vi "Tosca-Masker Thread.vi"(7 "IPC":T1, 11 "Tosca":refnum<class "Parameters.lvclass">) -> (0 "error out":errorcluster)   [LabVIEW 2020]
uses:
  IPC VIs/Tosca-IPC.ctl
  Classes/Parameters/Parameters.lvclass
  Digital Input VIs/Tosca-DI Queue Data.ctl
  Digital Input VIs/Tosca-Input Event.ctl
  Digital Input VIs/Tosca-Input Criterion.ctl
  epl-vi-lib/Utility VIs/Type Defs/Logic State.ctl
  Typedefs/Tosca-Accumulator.ctl
  Typedefs/Tosca-State AODO.ctl
  Typedefs/Tosca-AO Runtime.ctl
  Typedefs/Tosca-DO Runtime.ctl
  epl-vi-lib/Signal Synthesis VIs/4th Generation/Classes/SignalManager/SignalManager.lvclass
  Typedefs/Tosca-Synapse Start Data.ctl
  IPC VIs/Tosca-Message.ctl
  IPC VIs/Tosca-Message Action.ctl
  Typedefs/Tosca-Thread Type.ctl
  Imaging VIs/Tosca-2P-Notifier Data.ctl
  Typedefs/Tosca-MATLAB Queue Data.ctl
  Visual Stim VIs/Tosca-Grating.ctl
  Visual Stim VIs/Tosca-Grating Type.ctl
  Typedefs/Tosca-File IO Notification.ctl
  Classes/Parameters/Parameters.lvclass/Parameters.ctl
  epl-vi-lib/Signal Synthesis VIs/4th Generation/Classes/Channel/Channel.lvclass/Channel.ctl
  epl-vi-lib/Signal Synthesis VIs/4th Generation/Classes/Level/Level.lvclass/Level.ctl
  05e3e8bd-c3cb-450d-bf27-de7c8e806e93.vi
  9dbdce7e-9137-4943-9ff0-cc94a39cad21.vi
  epl-vi-lib/Signal Synthesis VIs/4th Generation/Classes/Channel/Write Level Value.vi
  <vilib>/DAQmx/write.llb/DAQmx Write (Analog 1D DBL 1Chan NSamp).vi
  epl-vi-lib/Signal Synthesis VIs/4th Generation/Classes/Channel/Read Destination.vi
  Classes/Parameters/Read Use masker.vi
  Classes/Parameters/Read Masker.vi
  Classes/Parameters/Read DAQ.vi
  epl-vi-lib/Signal Synthesis VIs/4th Generation/Classes/Level/Write Level.vi
  epl-vi-lib/Utility VIs/Controls/Utilities-Wait.vi/89bc9713-8f2c-40bd-a11f-1c800a437687.vi
  Tosca-Globals.vi
  <vilib>/Utility/config.llb/Open Config Data.vi
  <vilib>/Utility/config.llb/Get Key Names.vi
  <vilib>/Utility/config.llb/Read Key.vi
  <vilib>/Utility/config.llb/Read Key (String).vi
  epl-vi-lib/Utility VIs/Array Manipulation VIs/String Array to Comma Separated String.vi
  <vilib>/Utility/error.llb/Error Cluster From Error Code.vi
  <vilib>/Utility/config.llb/Close Config Data.vi
  <vilib>/DAQmx/miscellaneous.llb/DAQmx Fill In Error Info.vi
  <vilib>/Utility/High Resolution Polling Wait.vi
  epl-vi-lib/Signal Synthesis VIs/4th Generation/Classes/Channel/Channel.lvclass
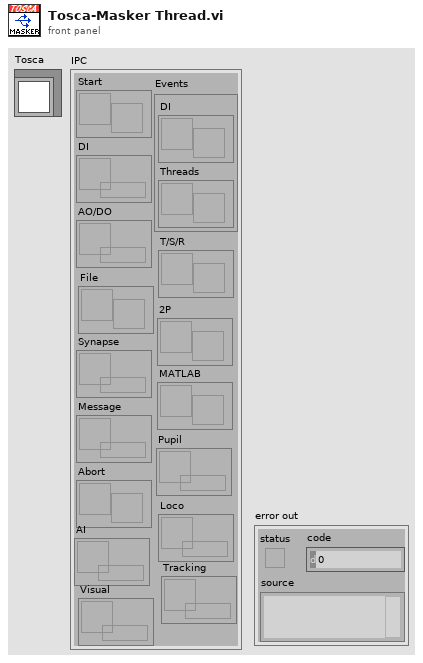
[diagram p1: front panel]
types:
  T1 = typedef "Tosca-IPC.ctl" = cluster{"Start":refnum<notifier>, "DI":refnum<queue>, "AO/DO":refnum<queue>, "Synapse":refnum<queue>, "Message":refnum<queue>, "Abort":refnum<notifier>, "Events":cluster{"DI":refnum<user-event>, "Threads ":refnum<user-event>}, "T/S/R":refnum<notifier>, "2P":refnum<notifier>, "MATLAB":refnum<notifier>, "Pupil":refnum<queue>, "Loco":refnum<queue>, "AI":refnum<queue>, "Tracking":refnum<queue>, "Visual":refnum<queue>, "File":refnum<notifier>}
  T2 = typedef "Parameters.lvclass/DAQ.ctl" = cluster{"AO Fs (Hz)":dbl, "DO Fs (Hz)":dbl, "Poll Rate (Hz)":dbl, "Baseline (s)":dbl}
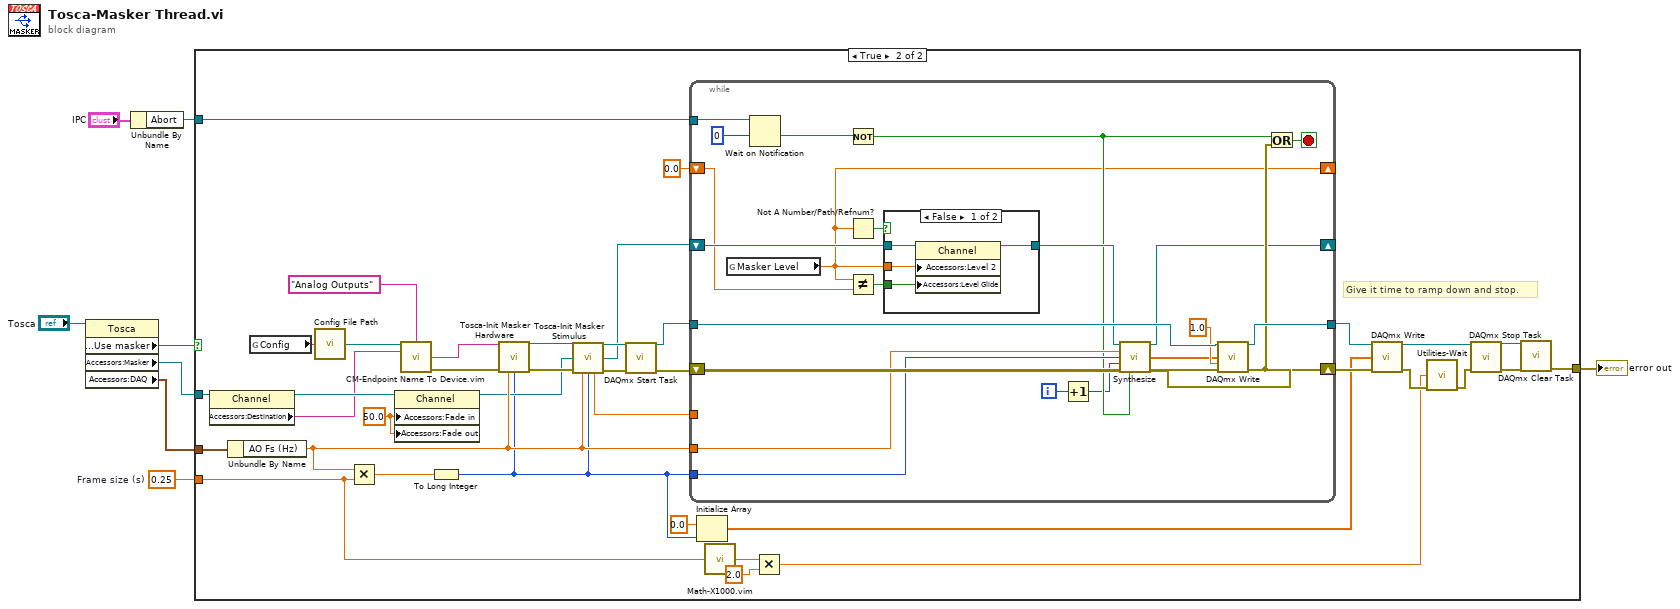
[diagram p0: block diagram]
diagram:
  w8 = 0.25  # Frame size (s)
  n1 = property class="Tosca"(reference="Tosca") -> ("Accessors:Use masker"=w3:bool, "Accessors:Masker"=w2:refnum<class "Channel.lvclass">, "Accessors:DAQ"=w1:T2)  [unwired: 1 in, 2 out]
  n2 = Unbundle By Name("IPC") -> ("Abort"=w5:refnum<notifier>)
  n3 = case shown="True" w3 {
    tunnel: w8 -> [_ w12]
    tunnel: [_ w37] -> w7
    tunnel: w5 -> [_ w35]
    tunnel: w2 -> [_ w33]
    tunnel: w1 -> [_ w32]
    frame False {
    }
    frame True {
      w27 = 50.0 ("Fade in")
      # "Give it time to ramp down and stop."
      n4 = property class="Channel"(reference=w33) -> (reference out=w30:refnum<class "Channel.lvclass">, "Accessors:Destination"=w24:string)  [unwired: 1 in, 1 out]
      n5 = Unbundle By Name(w32) -> ("AO Fs (Hz)"=w31:dbl)
      n6 = global read "Tosca-Globals.vi" "Config"() -> (w34:string)
      n7 = call "Config File Path.vi"("AppName"=w34) -> ("Default config file name"=w26:path)
      n8 = Multiply(x=w31, y=w12) -> (x*y=w46:dbl)
      n9 = property class="Channel"(reference=w30, "Accessors:Fade in"=w27, "Accessors:Fade out"=w27) -> (reference out=w28:refnum<class "Channel.lvclass">)  [unwired: 1 in, 1 out]
      n10 = call "CM-Endpoint Name To Device.vim"("Path"=w26, "IO Type"="Analog Outputs", "Names in"=w24) -> ("Devices"=w23:string, "error out"=w25:errorcluster)  [unwired: 9 in, 2 out]
      n11 = To Long Integer(number=w46) -> (32bit integer=w17:i32)
      n12 = call "Tosca-Init Masker Hardware.vi"("Channel"=w23, "error in (no error)"=w25, "Sampling rate (Hz)"=w31, "Npts"=w17) -> ("task out"=w44:refnum<k21>, "error out"=w45:errorcluster)  [unwired: 10 in]
      n13 = call "Tosca-Init Masker Stimulus.vi"("task in"=w44, "Channel"=w28, "error in (no error)"=w45, "Sampling rate (Hz)"=w31, "Npts"=w17) -> ("task out"=w36:refnum<k21>, "Channel out"=w29:refnum<class "Channel.lvclass">, "Ramp (ms)"=w38:dbl, "error out"=w39:errorcluster)  [unwired: 7 in]
      n14 = call <vilib>:"DAQmx Start Task.vi"("task/channels in"=w36, "error in"=w39) -> ("task out"=w40:refnum<k21>, "error out"=w41:errorcluster)  [unwired: 12 in]
      n15 = while {
        tunnel: w40 -> [w65]
        tunnel: [w67] -> w19
        shift-right: [w59] -> _
        shift-left: w29 -> [w68]
        tunnel: w31 -> [w55]
        tunnel: w17 -> [w56]
        tunnel: w38 -> [_]
        tunnel: w35 -> [w60]
        shift-right: [w62] -> w20
        shift-left: w41 -> [w69]
        shift-right: [w49] -> _
        shift-left: 0.0 ("Masker Level") -> [w50]
        i -> [w51]
        stop <- w66 stop-if-true
        n16 = global read "Tosca-Globals.vi" "Masker Level"() -> (w49:dbl)
        n17 = Wait on Notification(notifier=w60, timeout in ms (-1)=0) -> (timed out?=w53:bool)  [unwired: 2 in, 3 out]
        n18 = Not(x=w53) -> (.not. x?=w52:bool)
        n19 = Not A Number/Path/Refnum?(number/path/refnum=w49) -> (NaN/Path/Refnum?=w61:bool)
        n20 = Not Equal?(x=w49, y=w50) -> (x != y?=w48:bool)
        n21 = case shown="False" w61 {
          tunnel: w68 -> [w73 w74]
          tunnel: [w72 w74] -> w58
          tunnel: w49 -> [w71 _]
          tunnel: w48 -> [w70 _]
          frame False {
            n22 = property class="Channel"(reference=w73, "Accessors:Level 2"=w71, "Accessors:Level Glide"=w70) -> (reference out=w72:refnum<class "Channel.lvclass">)  [unwired: 1 in, 1 out]
          }
          frame True {
          }
        }
        n23 = Increment(x=w51) -> (x+1=w47:i32)
        n24 = call "Synthesize.vi"("Channel in"=w58, "Fs (Hz)"=w55, "Npts"=w56, "Repetition"=w47, "error in (no error)"=w69, "last"=w52) -> ("Channel out"=w59:refnum<class "Channel.lvclass">, "Array"=w57:dbl[], "error out"=w64:errorcluster)  [unwired: 6 in, 1 out]
        n25 = call-poly <vilib>:"DAQmx Write.vi"("task/channels in"=w65, "data"=w57, "timeout"=1.0, "error in"=w64) -> ("task out"=w67:refnum<k21>, "error out"=w62:errorcluster)  [unwired: 9 in, 1 out]
        n26 = Or(x=w52, y=w62) -> (x .or. y?=w66:bool)
      }
      n27 = Initialize Array(0.0 ("element"), w17) -> (w15:dbl[])
      n28 = call "Math-X1000.vim"("X"=w12) -> ("1000X"=w11:dbl)
      n29 = Multiply(x=w11, y=2.0) -> (x*y=w10:dbl)
      n30 = call-poly <vilib>:"DAQmx Write.vi"("task/channels in"=w19, "data"=w15, "error in"=w20) -> ("task out"=w18:refnum<k21>, "error out"=w13:errorcluster)  [unwired: 10 in, 1 out]
      n31 = call "Utilities-Wait.vi"("milliseconds to wait"=w10, "error in (no error)"=w13) -> ("error out"=w14:errorcluster)  [unwired: 13 in]
      n32 = call <vilib>:"DAQmx Stop Task.vi"("task/channels in"=w18, "error in"=w14) -> ("task out"=w43:refnum<k21>, "error out"=w42:errorcluster)  [unwired: 12 in]
      n33 = call <vilib>:"DAQmx Clear Task.vi"("task in"=w43, "error in"=w42) -> ("error out"=w37:errorcluster)  [unwired: 13 in]
    }
  }
  "error out" <- w7
